vi "Test - Draw Teapot.vi"() -> ()   [LabVIEW 2022 SP3, in "Raster.lvlib"] (continued)
, "UV"={"u"=0.0, "v"=0.0}, "Colour"=12517256}, "Alpha"=0.0, "Alpha Blending Enabled"=FALSE, "Colour"=5599805}, {"Vertex 1"={"Position"={"x"=400.0, "y"=248.05318, "z"=0.98371255}, "UV"={"u"=0.0, "v"=0.0}, "Colour"=12517256}, "Vertex 2"={"Position"={"x"=400.0, "y"=222.63887, "z"=0.98353577}, "UV"={"u"=0.0, "v"=0.0}, "Colour"=12517256}, "Vertex 3"={"Position"={"x"=344.93683, "y"=223.28236, "z"=0.9836732}, "UV"={"u"=0.0, "v"=0.0}, "Colour"=12517256}, "Alpha"=0.0, "Alpha Blending Enabled"=FALSE, "Colour"=10540915}, {"Vertex 1"={"Position"={"x"=346.02576, "y"=135.72502, "z"=0.9837993}, "UV"={"u"=0.0, "v"=0.0}, "Colour"=12517256}, "Vertex 2"={"Position"={"x"=344.29382, "y"=153.40399, "z"=0.9835987}, "UV"={"u"=0.0, "v"=0.0}, "Colour"=12517256}, "Vertex 3"={"Position"={"x"=400.0, "y"=152.15985, "z"=0.9834591}, "UV"={"u"=0.0, "v"=0.0}, "Colour"=12517256}, "Alpha"=0.0, "Alpha Blending Enabled"=FALSE, "Colour"=5599805}, {"Vertex 1"={"Position"={"x"=343.98178, "y"=198.56883, "z"=0.9835626}, "UV"={"u"=0.0, "v"=0.0}, "Colour"=12517256}, "Vertex 2"={"Position"={"x"=344.93683, "y"=223.28236, "z"=0.9836732}, "UV"={"u"=0.0, "v"=0.0}, "Colour"=12517256}, "Vertex 3"={"Position"={"x"=400.0, "y"=222.63887, "z"=0.98353577}, "UV"={"u"=0.0, "v"=0.0}, "Colour"=12517256}, "Alpha"=0.0, "Alpha Blending Enabled"=FALSE, "Colour"=10013805}, {"Vertex 1"={"Position"={"x"=400.0, "y"=134.37457, "z"=0.9836657}, "UV"={"u"=0.0, "v"=0.0}, "Colour"=12517256}, "Vertex 2"={"Position"={"x"=400.0, "y"=152.15985, "z"=0.9834591}, "UV"={"u"=0.0, "v"=0.0}, "Colour"=12517256}, "Vertex 3"={"Position"={"x"=455.7062, "y"=153.40399, "z"=0.9835987}, "UV"={"u"=0.0, "v"=0.0}, "Colour"=12517256}, "Alpha"=0.0, "Alpha Blending Enabled"=FALSE, "Colour"=5599805}, {"Vertex 1"={"Position"={"x"=455.0632, "y"=223.28236, "z"=0.9836732}, "UV"={"u"=0.0, "v"=0.0}, "Colour"=12517256}, "Vertex 2"={"Position"={"x"=456.01822, "y"=198.56883, "z"=0.9835626}, "UV"={"u"=0.0, "v"=0.0}, "Colour"=12517256}, "Vertex 3"={"Position"={"x"=400.0, "y"=197.70311, "z"=0.9834219}, "UV"={"u"=0.0, "v"=0.0}, "Colour"=12517256}, "Alpha"=0.0, "Alpha Blending Enabled"=FALSE, "Colour"=10013805}, {"Vertex 1"={"Position"={"x"=400.0, "y"=197.70311, "z"=0.9834219}, "UV"={"u"=0.0, "v"=0.0}, "Colour"=12517256}, "Vertex 2"={"Position"={"x"=400.0, "y"=222.63887, "z"=0.98353577}, "UV"={"u"=0.0, "v"=0.0}, "Colour"=12517256}, "Vertex 3"={"Position"={"x"=455.0632, "y"=223.28236, "z"=0.9836732}, "UV"={"u"=0.0, "v"=0.0}, "Colour"=12517256}, "Alpha"=0.0, "Alpha Blending Enabled"=FALSE, "Colour"=10013805}, {"Vertex 1"={"Position"={"x"=456.35504, "y"=174.77179, "z"=0.9835236}, "UV"={"u"=0.0, "v"=0.0}, "Colour"=12517256}, "Vertex 2"={"Position"={"x"=455.7062, "y"=153.40399, "z"=0.9835987}, "UV"={"u"=0.0, "v"=0.0}, "Colour"=12517256}, "Vertex 3"={"Position"={"x"=400.0, "y"=152.15985, "z"=0.9834591}, "UV"={"u"=0.0, "v"=0.0}, "Colour"=12517256}, "Alpha"=0.0, "Alpha Blending Enabled"=FALSE, "Colour"=7839573}, {"Vertex 1"={"Position"={"x"=400.0, "y"=222.63887, "z"=0.98353577}, "UV"={"u"=0.0, "v"=0.0}, "Colour"=12517256}, "Vertex 2"={"Position"={"x"=400.0, "y"=197.70311, "z"=0.9834219}, "UV"={"u"=0.0, "v"=0.0}, "Colour"=12517256}, "Vertex 3"={"Position"={"x"=343.98178, "y"=198.56883, "z"=0.9835626}, "UV"={"u"=0.0, "v"=0.0}, "Colour"=12517256}, "Alpha"=0.0, "Alpha Blending Enabled"=FALSE, "Colour"=10013805}, {"Vertex 1"={"Position"={"x"=343.64493, "y"=174.77179, "z"=0.9835236}, "UV"={"u"=0.0, "v"=0.0}, "Colour"=12517256}, "Vertex 2"={"Position"={"x"=343.98178, "y"=198.56883, "z"=0.9835626}, "UV"={"u"=0.0, "v"=0.0}, "Colour"=12517256}, "Vertex 3"={"Position"={"x"=400.0, "y"=197.70311, "z"=0.9834219}, "UV"={"u"=0.0, "v"=0.0}, "Colour"=12517256}, "Alpha"=0.0, "Alpha Blending Enabled"=FALSE, "Colour"=9289061}, {"Vertex 1"={"Position"={"x"=344.29382, "y"=153.40399, "z"=0.9835987}, "UV"={"u"=0.0, "v"=0.0}, "Colour"=12517256}, "Vertex 2"={"Position"={"x"=343.64493, "y"=174.77179, "z"=0.9835236}, "UV"={"u"=0.0, "v"=0.0}, "Colour"=12517256}, "Vertex 3"={"Position"={"x"=400.0, "y"=173.69646, "z"=0.9833816}, "UV"={"u"=0.0, "v"=0.0}, "Colour"=12517256}, "Alpha"=0.0, "Alpha Blending Enabled"=FALSE, "Colour"=7839573}, {"Vertex 1"={"Position"={"x"=456.01822, "y"=198.56883, "z"=0.9835626}, "UV"={"u"=0.0, "v"=0.0}, "Colour"=12517256}, "Vertex 2"={"Position"={"x"=456.35504, "y"=174.77179, "z"=0.9835236}, "UV"={"u"=0.0, "v"=0.0}, "Colour"=12517256}, "Vertex 3"={"Position"={"x"=400.0, "y"=173.69646, "z"=0.9833816}, "UV"={"u"=0.0, "v"=0.0}, "Colour"=12517256}, "Alpha"=0.0, "Alpha Blending Enabled"=FALSE, "Colour"=9289061}, {"Vertex 1"={"Position"={"x"=400.0, "y"=173.69646, "z"=0.9833816}, "UV"={"u"=0.0, "v"=0.0}, "Colour"=12517256}, "Vertex 2"={"Position"={"x"=400.0, "y"=152.15985, "z"=0.9834591}, "UV"={"u"=0.0, "v"=0.0}, "Colour"=12517256}, "Vertex 3"={"Position"={"x"=344.29382, "y"=153.40399, "z"=0.9835987}, "UV"={"u"=0.0, "v"=0.0}, "Colour"=12517256}, "Alpha"=0.0, "Alpha Blending Enabled"=FALSE, "Colour"=7839573}, {"Vertex 1"={"Position"={"x"=400.0, "y"=173.69646, "z"=0.9833816}, "UV"={"u"=0.0, "v"=0.0}, "Colour"=12517256}, "Vertex 2"={"Position"={"x"=400.0, "y"=197.70311, "z"=0.9834219}, "UV"={"u"=0.0, "v"=0.0}, "Colour"=12517256}, "Vertex 3"={"Position"={"x"=456.01822, "y"=198.56883, "z"=0.9835626}, "UV"={"u"=0.0, "v"=0.0}, "Colour"=12517256}, "Alpha"=0.0, "Alpha Blending Enabled"=FALSE, "Colour"=9289061}, {"Vertex 1"={"Position"={"x"=400.0, "y"=152.15985, "z"=0.9834591}, "UV"={"u"=0.0, "v"=0.0}, "Colour"=12517256}, "Vertex 2"={"Position"={"x"=400.0, "y"=173.69646, "z"=0.9833816}, "UV"={"u"=0.0, "v"=0.0}, "Colour"=12517256}, "Vertex 3"={"Position"={"x"=456.35504, "y"=174.77179, "z"=0.9835236}, "UV"={"u"=0.0, "v"=0.0}, "Colour"=12517256}, "Alpha"=0.0, "Alpha Blending Enabled"=FALSE, "Colour"=7839573}, {"Vertex 1"={"Position"={"x"=400.0, "y"=197.70311, "z"=0.9834219}, "UV"={"u"=0.0, "v"=0.0}, "Colour"=12517256}, "Vertex 2"={"Position"={"x"=400.0, "y"=173.69646, "z"=0.9833816}, "UV"={"u"=0.0, "v"=0.0}, "Colour"=12517256}, "Vertex 3"={"Position"={"x"=343.64493, "y"=174.77179, "z"=0.9835236}, "UV"={"u"=0.0, "v"=0.0}, "Colour"=12517256}, "Alpha"=0.0, "Alpha Blending Enabled"=FALSE, "Colour"=9289061}] {"Vertex 3"."UV"."v" min=0 max=1 step=0.1; "Vertex 3"."UV"."u" min=0 max=1 step=0.1; "Vertex 2"."UV"."v" min=0 max=1 step=0.1; "Vertex 2"."UV"."u" min=0 max=1 step=0.1; "Vertex 1"."UV"."v" min=0 max=1 step=0.1; "Vertex 1"."UV"."u" min=0 max=1 step=0.1}
  out "Time [s]":dbl format="%.3p"
  out "new picture":picture
  # "(0,0)"
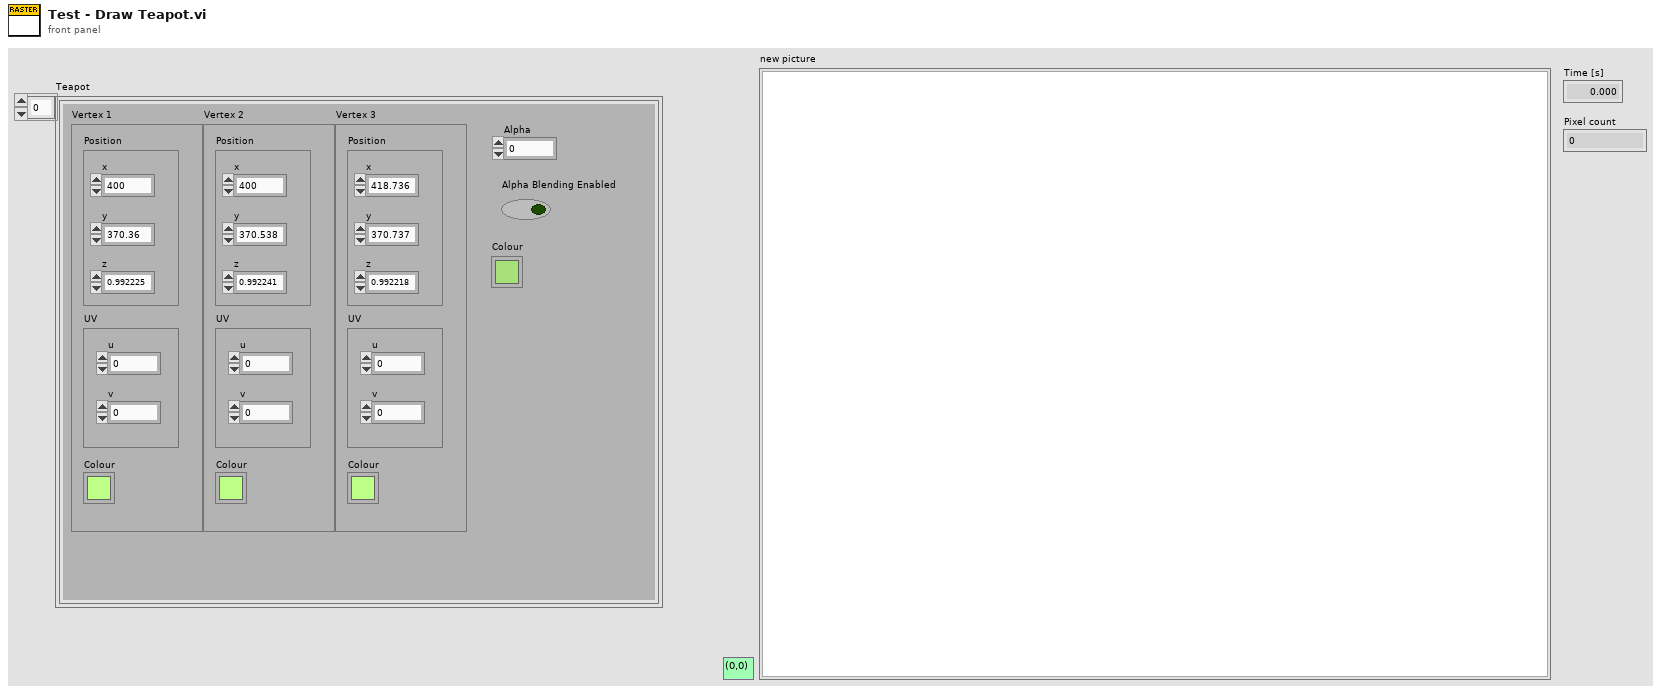
[diagram p1: front panel]
types:
  T1 = typedef "3D.lvlib/Triangle.ctl" = cluster{"Vertex 1":T2, "Vertex 2":T2, "Vertex 3":T2, "Alpha":dbl, "Alpha Blending Enabled":bool, "Colour":u32}
  T2 = typedef "3D.lvlib/Vertex.ctl" = cluster{"Position":T3, "UV":T4, "Colour":u32}
  T3 = typedef "3D.lvlib/Vector 3D.ctl" = cluster{"x":sgl, "y":sgl, "z":sgl}
  T4 = typedef "Raster.lvlib/UV.ctl" = cluster{"u":sgl, "v":sgl}
  T5 = typedef "Raster.lvlib/Rectangle Dimensions.ctl" = cluster{"Width":u32, "Height":u32}
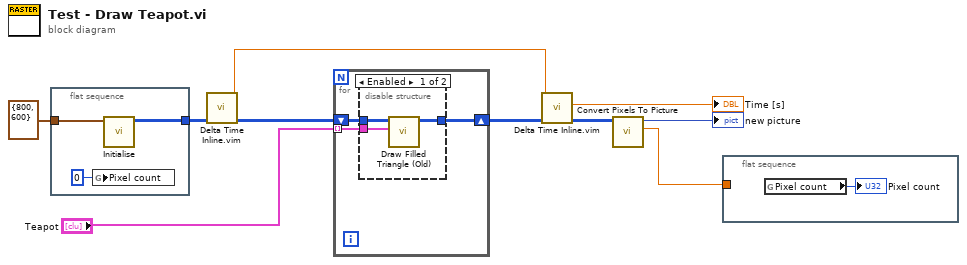
[diagram p0: block diagram]
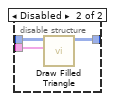
[diagram p2: hidden frame]
diagram:
  n1 = flat-sequence {
    tunnel: T5 {"Width"=800, "Height"=600} ("Screen Dimensions") -> [w13]
    tunnel: [w12] -> w8
    frame #0 {
      n2 = global write "Global 1.vi" "Pixel count"(u32 0 ("Pixel count")) -> ()
      n3 = call "Initialise.vi"("Screen Dimensions"=w13) -> ("Pixel Data out"=w12:u32[][])  [unwired: 10 in]
    }
  }
  n4 = call "Delta Time Inline.vim"("value in"=w8) -> ("value out"=w7:u32[][], "Relative Seconds out [s]"=w3:dbl)  [unwired: 8 in, 1 out]
  n5 = for {
    tunnel: "Teapot" -> [w14] mode=indexing
    shift-right: [w15] -> w6
    shift-left: w7 -> [w16]
    n6 = disable-structure shown="Enabled" {
      disable-tunnel: w16 -> [w19 w22]
      disable-tunnel: [w18 w21] -> w15
      disable-tunnel: w14 -> [w17 w20]
      frame Enabled {
        n7 = call "Draw Filled Triangle (Old).vi"("Triangle"=w17, "Pixel Data in"=w19) -> ("Pixel Data out"=w18:u32[][])  [unwired: 9 in]
      }
      frame Disabled {
        n8 = call "Draw Filled Triangle.vi"("Triangle"=w20, "Pixel Data in"=w22) -> ("Pixel Data out"=w21:u32[][])  [unwired: 9 in]
      }
    }
  }
  n9 = call "Delta Time Inline.vim"("value in"=w6, "Relative Seconds in [s]"=w3) -> ("value out"=w5:u32[][], "Delta Time [s]"=→"Time [s]":dbl)  [unwired: 7 in, 1 out]
  n10 = call "Convert Pixels To Picture.vi"("Pixel Data in"=w5) -> ("Present Time [s]"=w1:dbl, "2D Picture"=→"new picture":picture)  [unwired: 9 in]
  n11 = flat-sequence {
    tunnel: w1 -> [_]
    frame #0 {
      n12 = global read "Global 1.vi" "Pixel count"() -> (→"Pixel count":u32)
    }
  }
